vi "CLEAN CR LF.vi"(8 "errin":errorcluster, 11 "in":string) -> (0 "errout":errorcluster, 3 "out":string)   [LabVIEW 2020]
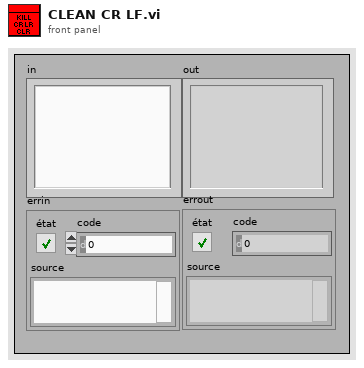
[diagram p1: front panel]
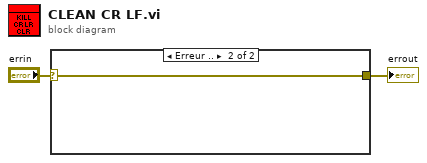
[diagram p0: block diagram]
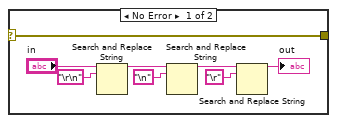
[diagram p2: hidden frame]
diagram:
  n1 = case shown="Erreur .." "errin" {
    selector: "errin" -> [w3 w11]
    tunnel: [w3 w11] -> w1
    frame No Error {
      n2 = Search and Replace String(input string="in", search string="\r\n") -> (result string=w8:string)  [unwired: 6 in, 3 out]
      n3 = Search and Replace String(input string=w8, search string="\n") -> (result string=w7:string)  [unwired: 6 in, 3 out]
      n4 = Search and Replace String(input string=w7, search string="\r") -> (result string=→"out":string)  [unwired: 6 in, 3 out]
    }
    frame Error {
    }
  }
  "errout" <- w1
